vi "sema-need-why.vi"() -> ()   [LabVIEW 2013]
panel:
  out "C":bool
  out "B":bool
  out "A":bool
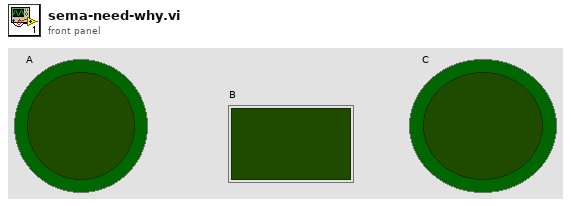
[diagram p1: front panel]
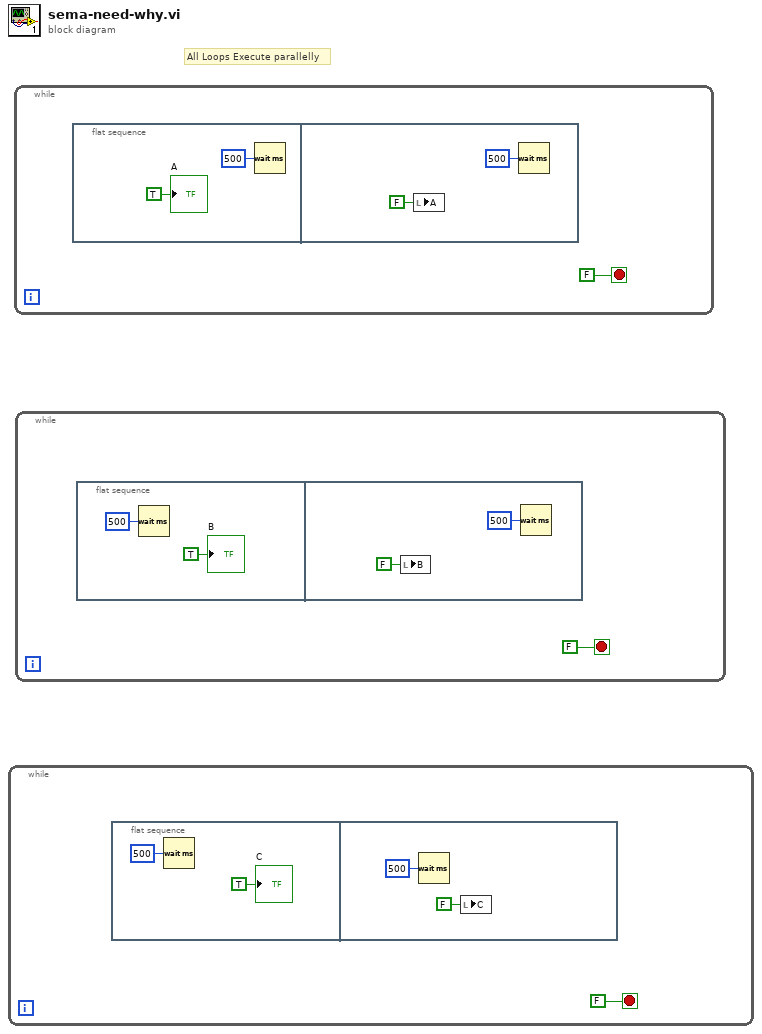
[diagram p0: block diagram]
diagram:
  # "All Loops Execute parallelly"
  n1 = while {
    stop <- FALSE stop-if-true
    n2 = flat-sequence {
      frame #0 {
        n3 = Wait (ms)(milliseconds to wait=u32 500) -> ()  [unwired: 1 out]
        "C" <- TRUE ("C")
      }
      frame #1 {
        n4 = Wait (ms)(milliseconds to wait=u32 500) -> ()  [unwired: 1 out]
        n5 = local write "C"(FALSE ("C")) -> ()
      }
    }
  }
  n6 = while {
    stop <- FALSE stop-if-true
    n7 = flat-sequence {
      frame #0 {
        n8 = Wait (ms)(milliseconds to wait=u32 500) -> ()  [unwired: 1 out]
        "A" <- TRUE ("A")
      }
      frame #1 {
        n9 = local write "A"(FALSE ("A")) -> ()
        n10 = Wait (ms)(milliseconds to wait=u32 500) -> ()  [unwired: 1 out]
      }
    }
  }
  n11 = while {
    stop <- FALSE stop-if-true
    n12 = flat-sequence {
      frame #0 {
        n13 = Wait (ms)(milliseconds to wait=u32 500) -> ()  [unwired: 1 out]
        "B" <- TRUE ("B")
      }
      frame #1 {
        n14 = local write "B"(FALSE ("B")) -> ()
        n15 = Wait (ms)(milliseconds to wait=u32 500) -> ()  [unwired: 1 out]
      }
    }
  }
